vi "util-path-to-proc-name.vi"(10 "location (DIR_PROCS)":T1, 11 "File path":path) -> (3 "String":string)   [LabVIEW 2024]
uses:
  controls/typePathSelector.ctl
  <vilib>/Utility/error.llb/Clear Errors.vi
  <vilib>/Utility/libraryn.llb/Create Directory Recursive.vi
panel:
  out "array out":string[](array[string])
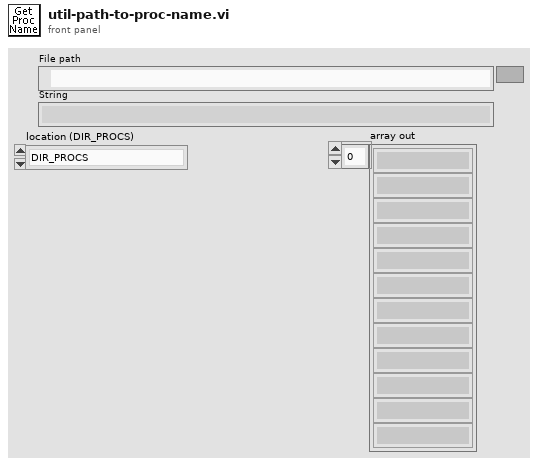
[diagram p1: front panel]
types:
  T1 = typedef "typePathSelector.ctl" = enum16{"DIR_PROCS", "DIR_CONFIG", "DIR_TEMPLATE", "DIR_IO_FILE", "DIR_RECORD", "DIR_LOG", "DIR_RUNTIME", "DIR_PRESET", "DIR_INI"}
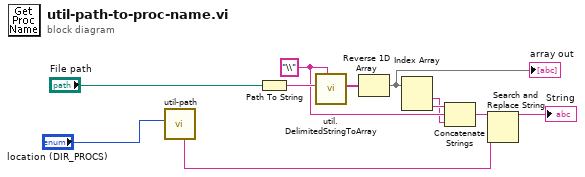
[diagram p0: block diagram]
diagram:
  w5 = "\\" ("delimiter (,)")
  n1 = call "util-path.vi"("Selected Folder (PROCS)"="location (DIR_PROCS)") -> (".extension (.prc)"=w3:string)  [unwired: 6 in, 4 out]
  n2 = Path To String(path="File path") -> (string=w9:string)
  n3 = call "util.DelimitedStringToArray.vi"("delimiter (,)"=w5, "delimitaed string"=w9) -> ("array out"=w8:string[])  [unwired: 9 in]
  n4 = Reverse 1D Array(array=w8) -> (reversed array=w7:string[])
  "array out" <- w7
  n5 = Index Array(array=w7) -> (element #1=w4:string, element #2=w6:string)  [unwired: 2 in]
  n6 = Concatenate Strings(w6, w5, w4) -> (w2:string)
  n7 = Search and Replace String(input string=w2, search string=w3) -> (result string=→"String":string)  [unwired: 6 in, 3 out]
